vi "Send_To_Dashboard.vi"   [LabVIEW 2018]
uses:
  Global_Variables/Sensor_Values.vi
  <vilib>/Rock Robotics/Network Tables/NT Write Number.vi
  <vilib>/Rock Robotics/Network Tables/NT Write Boolean.vi
  <vilib>/Rock Robotics/Network Tables/NT Write String.vi
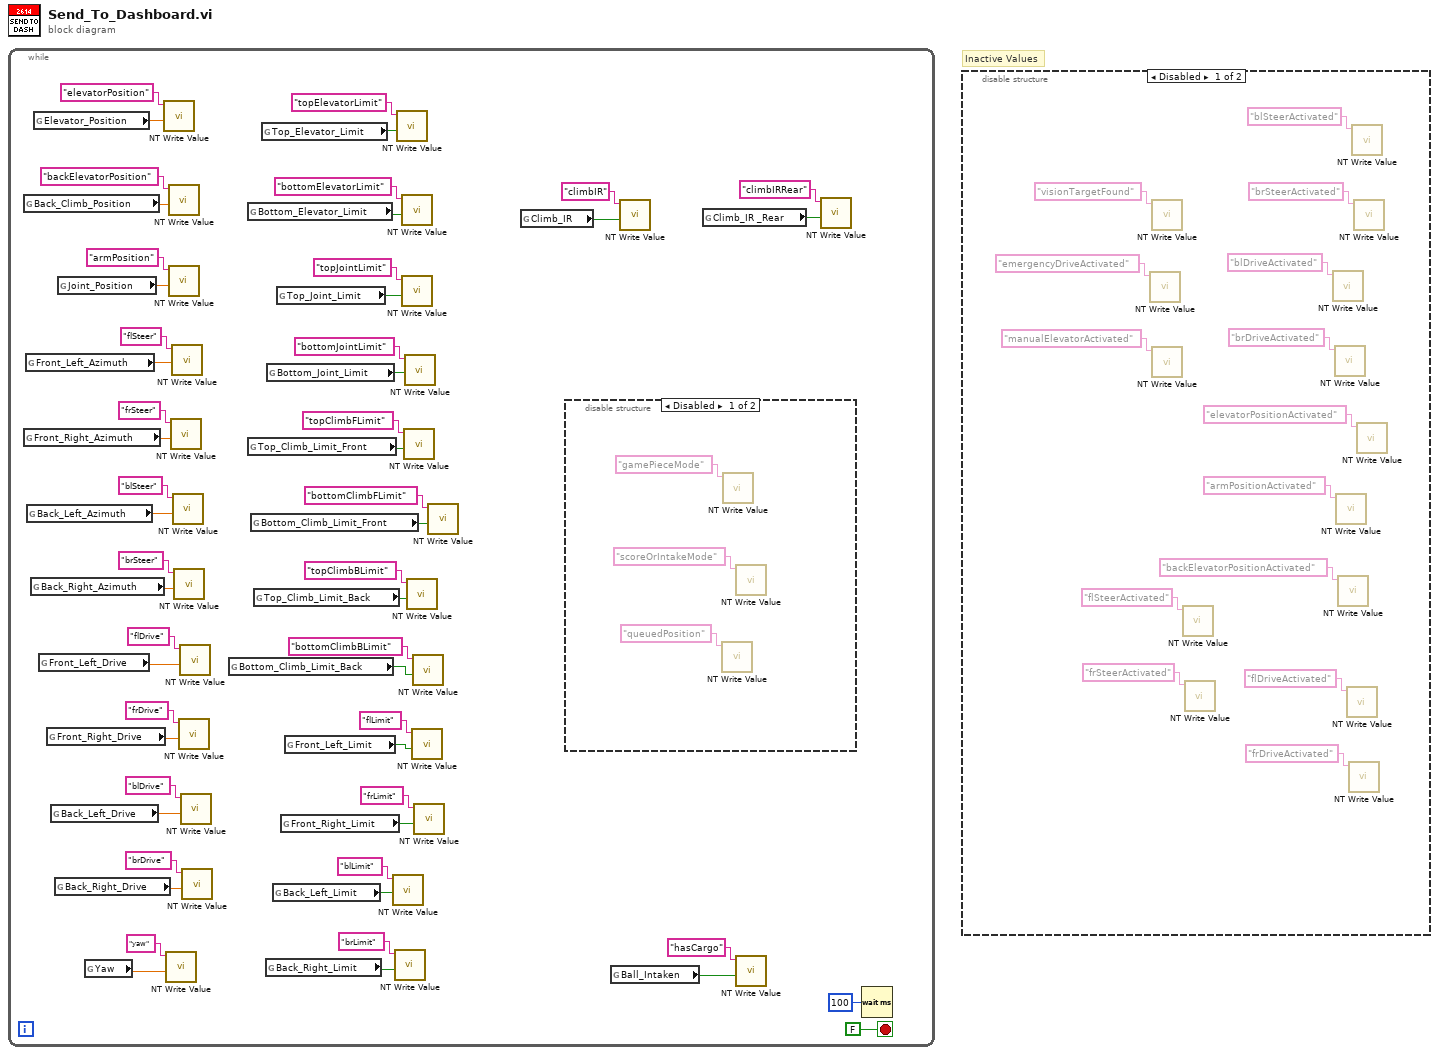
[diagram p0: block diagram]
diagram:
  # "Inactive Values"
  n1 = while {
    stop <- FALSE stop-if-true
    n2 = global read "Sensor_Values.vi" "Back_Climb_Position"() -> (w28:dbl)
    n3 = global read "Sensor_Values.vi" "Front_Right_Azimuth"() -> (w25:dbl)
    n4 = global read "Sensor_Values.vi" "Front_Left_Azimuth"() -> (w26:dbl)
    n5 = global read "Sensor_Values.vi" "Back_Left_Azimuth"() -> (w24:dbl)
    n6 = global read "Sensor_Values.vi" "Back_Right_Azimuth"() -> (w23:dbl)
    n7 = global read "Sensor_Values.vi" "Elevator_Position"() -> (w29:dbl)
    n8 = global read "Sensor_Values.vi" "Front_Left_Drive"() -> (w22:dbl)
    n9 = global read "Sensor_Values.vi" "Front_Right_Drive"() -> (w21:dbl)
    n10 = global read "Sensor_Values.vi" "Back_Left_Drive"() -> (w20:dbl)
    n11 = global read "Sensor_Values.vi" "Back_Right_Drive"() -> (w19:dbl)
    n12 = global read "Sensor_Values.vi" "Joint_Position"() -> (w27:dbl)
    n13 = global read "Sensor_Values.vi" "Yaw"() -> (w5:dbl)
    n14 = call-poly <vilib>:"NT Write Value.vi"("Numeric"=w29, "Name"="elevatorPosition") -> ()  [unwired: 9 in, 1 out]
    n15 = call-poly <vilib>:"NT Write Value.vi"("Numeric"=w5, "Name"="yaw") -> ()  [unwired: 9 in, 1 out]
    n16 = call-poly <vilib>:"NT Write Value.vi"("Numeric"=w28, "Name"="backElevatorPosition") -> ()  [unwired: 9 in, 1 out]
    n17 = call-poly <vilib>:"NT Write Value.vi"("Numeric"=w27, "Name"="armPosition") -> ()  [unwired: 9 in, 1 out]
    n18 = call-poly <vilib>:"NT Write Value.vi"("Numeric"=w25, "Name"="frSteer") -> ()  [unwired: 9 in, 1 out]
    n19 = call-poly <vilib>:"NT Write Value.vi"("Numeric"=w26, "Name"="flSteer") -> ()  [unwired: 9 in, 1 out]
    n20 = call-poly <vilib>:"NT Write Value.vi"("Numeric"=w24, "Name"="blSteer") -> ()  [unwired: 9 in, 1 out]
    n21 = call-poly <vilib>:"NT Write Value.vi"("Numeric"=w23, "Name"="brSteer") -> ()  [unwired: 9 in, 1 out]
    n22 = call-poly <vilib>:"NT Write Value.vi"("Numeric"=w21, "Name"="frDrive") -> ()  [unwired: 9 in, 1 out]
    n23 = call-poly <vilib>:"NT Write Value.vi"("Numeric"=w22, "Name"="flDrive") -> ()  [unwired: 9 in, 1 out]
    n24 = call-poly <vilib>:"NT Write Value.vi"("Numeric"=w20, "Name"="blDrive") -> ()  [unwired: 9 in, 1 out]
    n25 = call-poly <vilib>:"NT Write Value.vi"("Numeric"=w19, "Name"="brDrive") -> ()  [unwired: 9 in, 1 out]
    n26 = global read "Sensor_Values.vi" "Bottom_Climb_Limit_Back"() -> (w11:bool)
    n27 = global read "Sensor_Values.vi" "Bottom_Elevator_Limit"() -> (w17:bool)
    n28 = global read "Sensor_Values.vi" "Top_Climb_Limit_Front"() -> (w14:bool)
    n29 = global read "Sensor_Values.vi" "Bottom_Climb_Limit_Front"() -> (w13:bool)
    n30 = global read "Sensor_Values.vi" "Top_Climb_Limit_Back"() -> (w12:bool)
    n31 = global read "Sensor_Values.vi" "Top_Elevator_Limit"() -> (w18:bool)
    n32 = global read "Sensor_Values.vi" "Back_Right_Limit"() -> (w7:bool)
    n33 = global read "Sensor_Values.vi" "Bottom_Joint_Limit"() -> (w15:bool)
    n34 = global read "Sensor_Values.vi" "Back_Left_Limit"() -> (w8:bool)
    n35 = global read "Sensor_Values.vi" "Top_Joint_Limit"() -> (w16:bool)
    n36 = global read "Sensor_Values.vi" "Front_Right_Limit"() -> (w9:bool)
    n37 = global read "Sensor_Values.vi" "Front_Left_Limit"() -> (w10:bool)
    n38 = call-poly <vilib>:"NT Write Value.vi"("Boolean"=w8, "Name"="blLimit") -> ()  [unwired: 9 in, 1 out]
    n39 = call-poly <vilib>:"NT Write Value.vi"("Boolean"=w7, "Name"="brLimit") -> ()  [unwired: 9 in, 1 out]
    n40 = call-poly <vilib>:"NT Write Value.vi"("Boolean"=w18, "Name"="topElevatorLimit") -> ()  [unwired: 9 in, 1 out]
    n41 = call-poly <vilib>:"NT Write Value.vi"("Boolean"=w17, "Name"="bottomElevatorLimit") -> ()  [unwired: 9 in, 1 out]
    n42 = call-poly <vilib>:"NT Write Value.vi"("Boolean"=w16, "Name"="topJointLimit") -> ()  [unwired: 9 in, 1 out]
    n43 = call-poly <vilib>:"NT Write Value.vi"("Boolean"=w14, "Name"="topClimbFLimit") -> ()  [unwired: 9 in, 1 out]
    n44 = call-poly <vilib>:"NT Write Value.vi"("Boolean"=w15, "Name"="bottomJointLimit") -> ()  [unwired: 9 in, 1 out]
    n45 = call-poly <vilib>:"NT Write Value.vi"("Boolean"=w12, "Name"="topClimbBLimit") -> ()  [unwired: 9 in, 1 out]
    n46 = call-poly <vilib>:"NT Write Value.vi"("Boolean"=w10, "Name"="flLimit") -> ()  [unwired: 9 in, 1 out]
    n47 = call-poly <vilib>:"NT Write Value.vi"("Boolean"=w11, "Name"="bottomClimbBLimit") -> ()  [unwired: 9 in, 1 out]
    n48 = call-poly <vilib>:"NT Write Value.vi"("Boolean"=w9, "Name"="frLimit") -> ()  [unwired: 9 in, 1 out]
    n49 = call-poly <vilib>:"NT Write Value.vi"("Boolean"=w13, "Name"="bottomClimbFLimit") -> ()  [unwired: 9 in, 1 out]
    n50 = global read "Sensor_Values.vi" "Climb_IR"() -> (w2:bool)
    n51 = disable-structure shown="Disabled" {
      frame Disabled {
        n52 = call-poly <vilib>:"NT Write Value.vi"("Name"="queuedPosition") -> ()  [unwired: 10 in, 1 out]
        n53 = call-poly <vilib>:"NT Write Value.vi"("Name"="gamePieceMode") -> ()  [unwired: 10 in, 1 out]
        n54 = call-poly <vilib>:"NT Write Value.vi"("Name"="scoreOrIntakeMode") -> ()  [unwired: 10 in, 1 out]
      }
      frame Enabled {
      }
    }
    n55 = global read "Sensor_Values.vi" "Ball_Intaken"() -> (w6:bool)
    n56 = call-poly <vilib>:"NT Write Value.vi"("Boolean"=w2, "Name"="climbIR") -> ()  [unwired: 9 in, 1 out]
    n57 = global read "Sensor_Values.vi" "Climb_IR _Rear"() -> (w1:bool)
    n58 = call-poly <vilib>:"NT Write Value.vi"("Boolean"=w6, "Name"="hasCargo") -> ()  [unwired: 9 in, 1 out]
    n59 = call-poly <vilib>:"NT Write Value.vi"("Boolean"=w1, "Name"="climbIRRear") -> ()  [unwired: 9 in, 1 out]
    n60 = Wait (ms)(milliseconds to wait=u32 100) -> ()  [unwired: 1 out]
  }
  n61 = disable-structure shown="Disabled" {
    frame Disabled {
      n62 = call-poly <vilib>:"NT Write Value.vi"("Name"="emergencyDriveActivated") -> ()  [unwired: 10 in, 1 out]
      n63 = call-poly <vilib>:"NT Write Value.vi"("Name"="visionTargetFound") -> ()  [unwired: 10 in, 1 out]
      n64 = call-poly <vilib>:"NT Write Value.vi"("Name"="manualElevatorActivated") -> ()  [unwired: 10 in, 1 out]
      n65 = call-poly <vilib>:"NT Write Value.vi"("Name"="flSteerActivated") -> ()  [unwired: 10 in, 1 out]
      n66 = call-poly <vilib>:"NT Write Value.vi"("Name"="frSteerActivated") -> ()  [unwired: 10 in, 1 out]
      n67 = call-poly <vilib>:"NT Write Value.vi"("Name"="blDriveActivated") -> ()  [unwired: 10 in, 1 out]
      n68 = call-poly <vilib>:"NT Write Value.vi"("Name"="brDriveActivated") -> ()  [unwired: 10 in, 1 out]
      n69 = call-poly <vilib>:"NT Write Value.vi"("Name"="armPositionActivated") -> ()  [unwired: 10 in, 1 out]
      n70 = call-poly <vilib>:"NT Write Value.vi"("Name"="backElevatorPositionActivated") -> ()  [unwired: 10 in, 1 out]
      n71 = call-poly <vilib>:"NT Write Value.vi"("Name"="flDriveActivated") -> ()  [unwired: 10 in, 1 out]
      n72 = call-poly <vilib>:"NT Write Value.vi"("Name"="frDriveActivated") -> ()  [unwired: 10 in, 1 out]
      n73 = call-poly <vilib>:"NT Write Value.vi"("Name"="blSteerActivated") -> ()  [unwired: 10 in, 1 out]
      n74 = call-poly <vilib>:"NT Write Value.vi"("Name"="brSteerActivated") -> ()  [unwired: 10 in, 1 out]
      n75 = call-poly <vilib>:"NT Write Value.vi"("Name"="elevatorPositionActivated") -> ()  [unwired: 10 in, 1 out]
    }
    frame Enabled {
    }
  }
